vi "Parse NIC Info.vi"(6 "ifconfig":string="# This file describes the network interfaces available on your system\n# and how to activate them. For more information, see interfaces(5).\n\n# The loopback network interface\nauto lo\niface lo inet loopback\n\n# The primary network interface\n#auto eth0\n#iface eth0 inet dhcp\n# Example to keep MAC address between reboots\n#hwaddress ether DE:AD:BE:EF:CA:FE\n\n# The secondary network interface\n#auto eth1\n#iface eth1 inet dhcp\n\n# WiFi Example\n#auto wlan0\n#iface wlan0 inet dhcp\n#    wpa-ssid \"essid\"\n#    wpa-psk  \"password\"\n\n# Ethernet/RNDIS gadget (g_ether)\n# Used by: /opt/scripts/boot/autoconfigure_usb0.sh\niface usb0 inet static\n    address 192.168.7.2\n    netmask 255.255.255.252\n    network 192.168.7.0\n    gateway 192.168.7.1e", 8 "Error In":errorcluster, 9 "All NICs":string[](array[string]), 10 "interfaces config":string="# This file describes the network interfaces available on your system\n# and how to activate them. For more information, see interfaces(5).\n\n# The loopback network interface\nauto lo\niface lo inet loopback\n\n# The primary network interface\n#auto eth0\n#iface eth0 inet dhcp\n# Example to keep MAC address between reboots\n#hwaddress ether DE:AD:BE:EF:CA:FE\n\n# The secondary network interface\n#auto eth1\n#iface eth1 inet dhcp\n\n# WiFi Example\n#auto wlan0\n#iface wlan0 inet dhcp\n#    wpa-ssid \"essid\"\n#    wpa-psk  \"password\"\n\n# Ethernet/RNDIS gadget (g_ether)\n# Used by: /opt/scripts/boot/autoconfigure_usb0.sh\niface usb0 inet static\n    address 192.168.7.2\n    netmask 255.255.255.252\n    network 192.168.7.0\n    gateway 192.168.7.1e", 11 "Install LV Data":T1={"SSH Session"=refnum, "Status Log"="", "Detailed Log"="", "Credentials"={"Hostname or IP"="192.168.7.2", "Username"="root", "Password"=""}, "Target Info"={"OS Version"="", "CPU"="", "Systemd Version"="", "Internet Access"=FALSE, "Device Type"="", "LV Installed Ver"="", "LV Available Ver"="", "LV Upgrade Available"=FALSE, "Hostname"="", "NIC Info"=[]}, "Reboot Required?"=FALSE}) -> (0 "Error Out":errorcluster, 3 "Install LV Data":T1={"SSH Session"=refnum, "Status Log"="", "Detailed Log"="", "Credentials"={"Hostname or IP"="192.168.7.2", "Username"="root", "Password"=""}, "Target Info"={"OS Version"="", "CPU"="", "Systemd Version"="", "Internet Access"=FALSE, "Device Type"="", "LV Installed Ver"="", "LV Available Ver"="", "LV Upgrade Available"=FALSE, "Hostname"="", "NIC Info"=[]}, "Reboot Required?"=FALSE})   [LabVIEW 2014, in "LMH-LINX.lvlib"]
uses:
  <vilib>/MakerHub/LINX/LMH-LINX.lvlib
  <vilib>/MakerHub/LINX/Private/Utilties/Target Management/Install LV Data.ctl
  C:/Program Files (x86)/National Instruments/LabVIEW 2014/vi.lib/MakerHub/LINX/Resources/Renci.SshNet.dll
  Resources/Renci.SshNet.dll
  <vilib>/MakerHub/LINX/Private/Utilties/Target Management/Target Info.ctl
  <vilib>/MakerHub/LINX/Private/Utilties/Target Management/NIC Info.ctl
  <vilib>/MakerHub/LINX/Private/Utilties/Target Management/NIC Mode.ctl
  <vilib>/regexp/Match Regular Expression.xnode
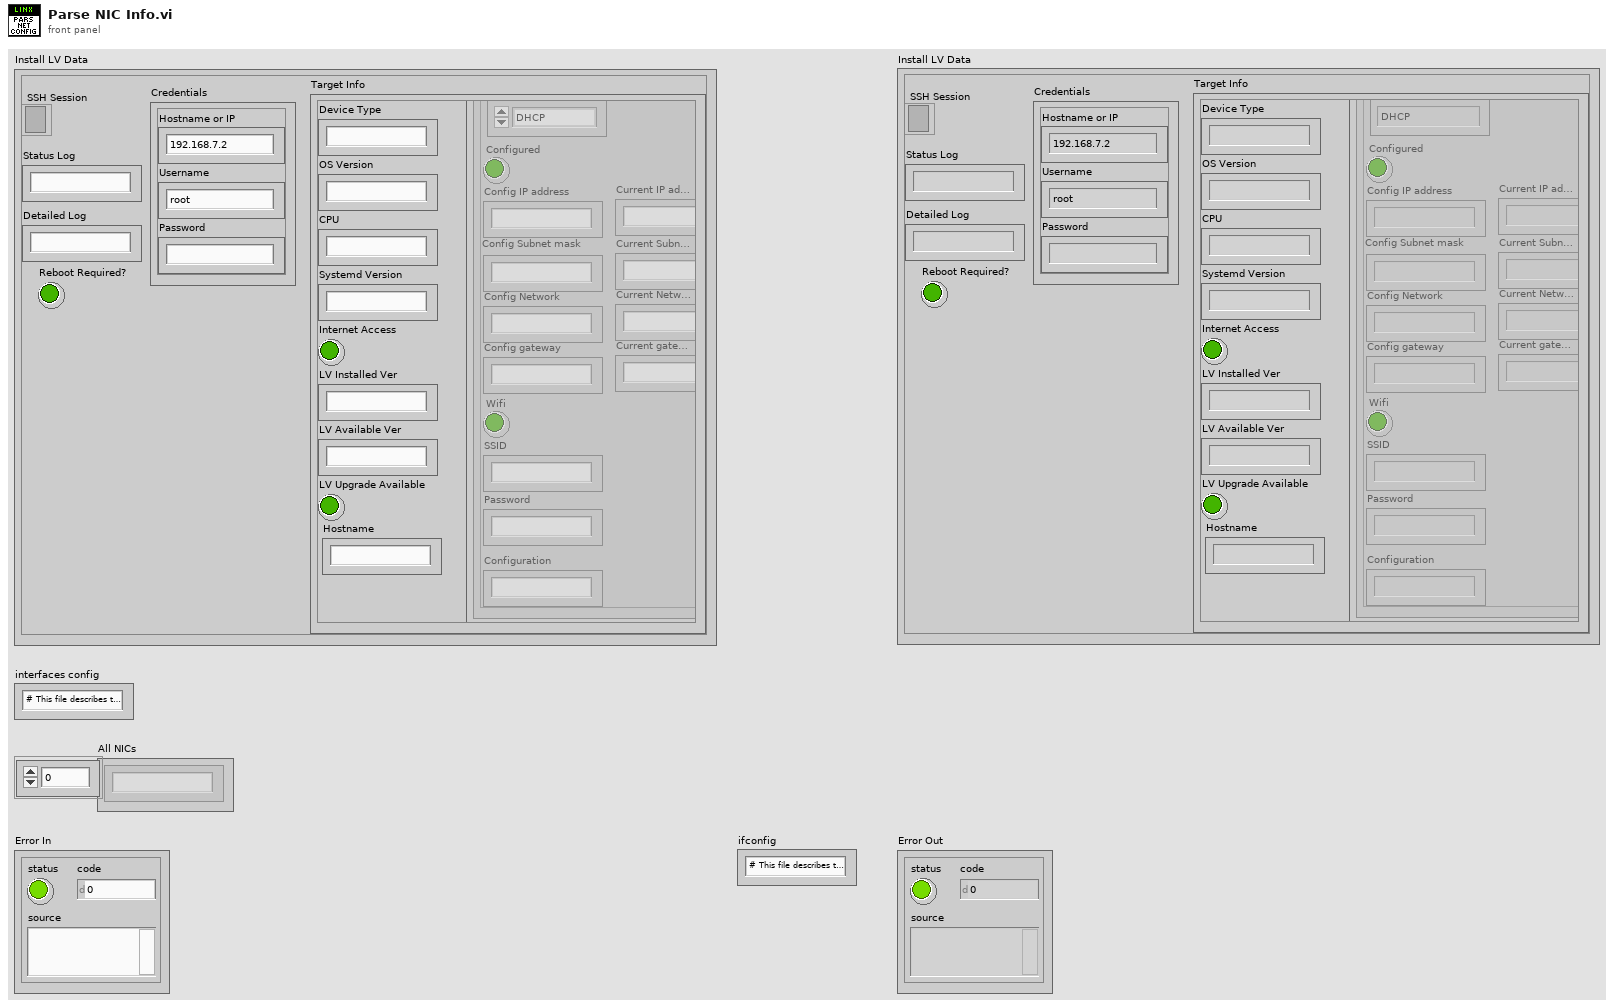
[diagram p1: front panel]
types:
  T1 = typedef "LMH-LINX.lvlib/Install LV Data.ctl" = cluster{"SSH Session":refnum<k24>, "Status Log":string, "Detailed Log":string, "Credentials":cluster{"Hostname or IP":string, "Username":string, "Password":string}, "Target Info":T2, "Reboot Required?":bool}
  T2 = typedef "LMH-LINX.lvlib/Target Info.ctl" = cluster{"OS Version":string, "CPU":string, "Systemd Version":string, "Internet Access":bool, "Device Type":string, "LV Installed Ver":string, "LV Available Ver":string, "LV Upgrade Available":bool, "Hostname":string, "NIC Info":T3[]}
  T3 = typedef "LMH-LINX.lvlib/NIC Info.ctl" = cluster{"Name":string, "NIC Mode":T4, "Configured":bool, "Config IP address":string, "Config Subnet mask":string, "Config Network":string, "Config gateway":string, "Wifi":bool, "SSID":string, "Password":string, "Configuration":string, "Current IP address":string, "Current Subnet mask":string, "Current gateway":string, "Current Network":string}
  T4 = typedef "LMH-LINX.lvlib/NIC Mode.ctl" = enum16{"DHCP", "Static", "Loopback"}
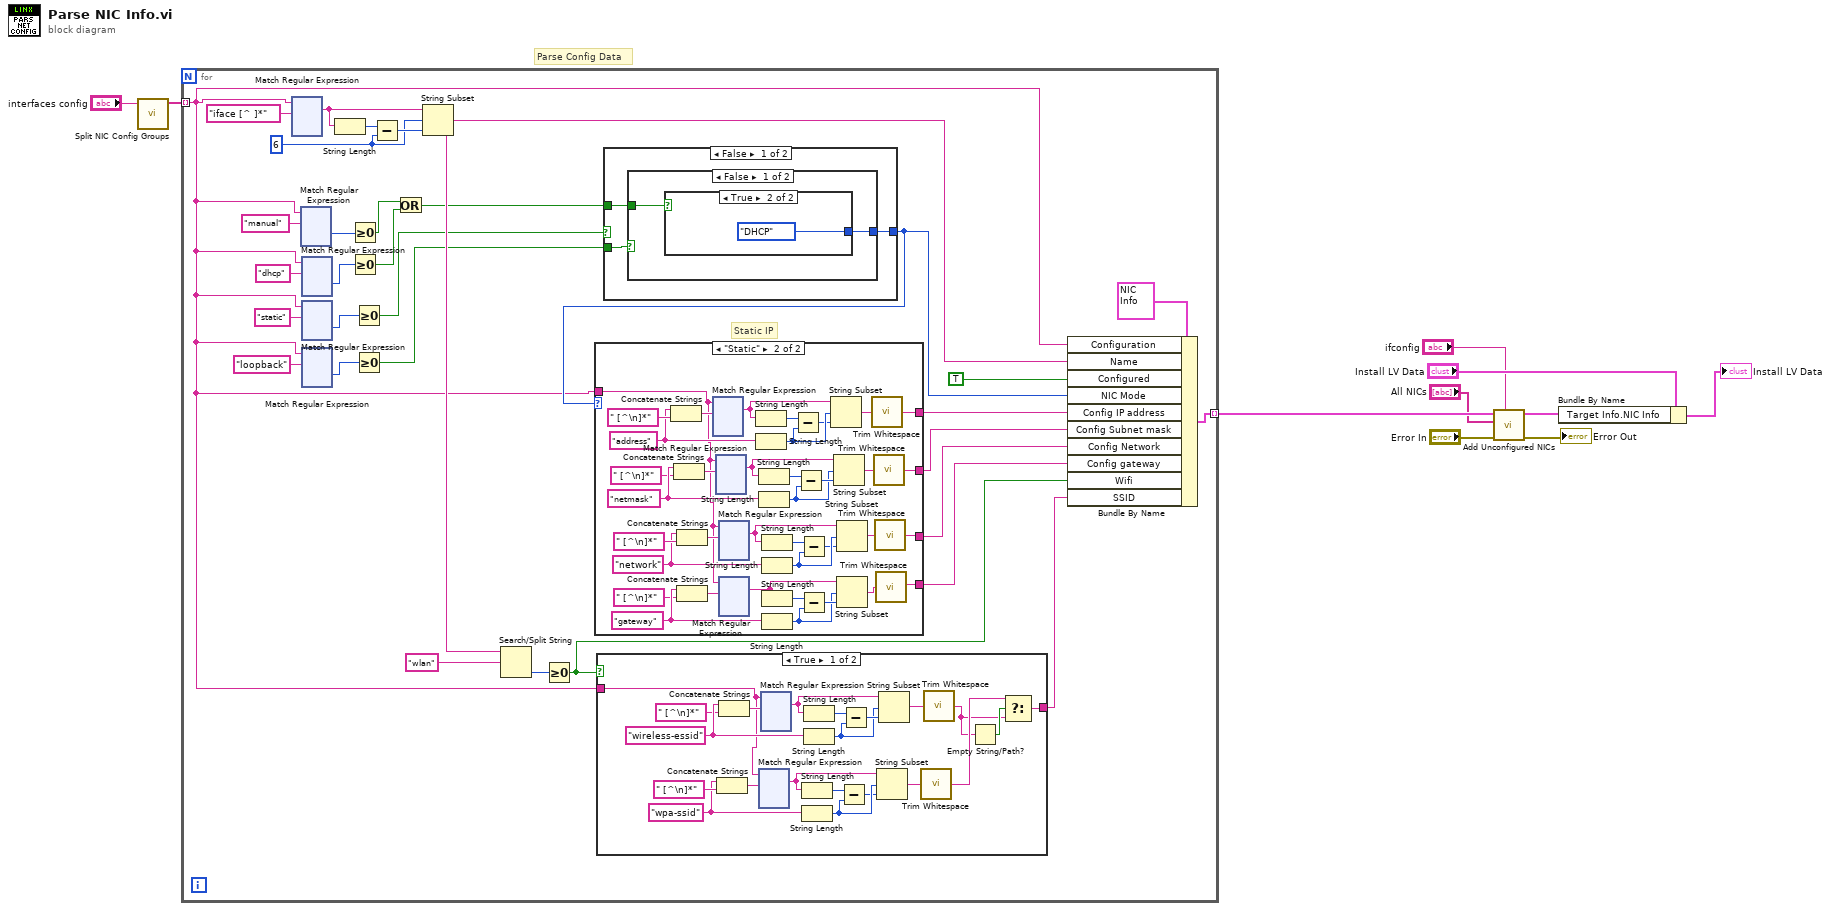
[diagram p0: block diagram]
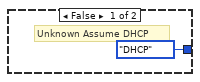
[diagram p2: hidden frame]
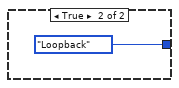
[diagram p3: hidden frame]
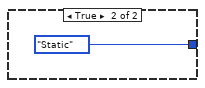
[diagram p4: hidden frame]
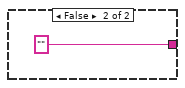
[diagram p5: hidden frame]
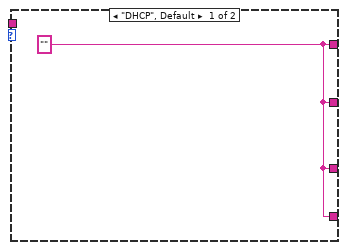
[diagram p6: hidden frame]
diagram:
  # "Parse Config Data"
  n1 = call <vilib>:"Split NIC Config Groups.vi"("Network Interface Config"="interfaces config") -> ("NIC Config Groups"=w9:string[])  [unwired: 10 in]
  n2 = for {
    tunnel: w9 -> [w12] mode=indexing
    tunnel: [w23] -> w6 mode=indexing
    w38 = 6 ("y")
    # "Static IP"
    n3 = xnode "Match Regular Expression"("input string"=w12, "regular expression"="iface [^ ]*") -> ("whole match"=w39:string)  [unwired: 4 in, 4 out]
    n4 = xnode "Match Regular Expression"("input string"=w12, "regular expression"="manual") -> ("offset past match"=w34:i32)  [unwired: 4 in, 4 out]
    n5 = xnode "Match Regular Expression"("input string"=w12, "regular expression"="dhcp") -> ("offset past match"=w32:i32)  [unwired: 4 in, 4 out]
    n6 = xnode "Match Regular Expression"("input string"=w12, "regular expression"="static") -> ("offset past match"=w33:i32)  [unwired: 4 in, 4 out]
    n7 = xnode "Match Regular Expression"("input string"=w12, "regular expression"="loopback") -> ("offset past match"=w20:i32)  [unwired: 4 in, 4 out]
    n8 = String Length(string=w39) -> (length=w41:i32)
    n9 = Greater Or Equal To 0?(x=w34) -> (x >= 0?=w16:bool)
    n10 = Greater Or Equal To 0?(x=w32) -> (x >= 0?=w15:bool)
    n11 = Greater Or Equal To 0?(x=w33) -> (x >= 0?=w18:bool)
    n12 = Greater Or Equal To 0?(x=w20) -> (x >= 0?=w17:bool)
    n13 = Subtract(x=w41, y=w38) -> (x-y=w40:i32)
    n14 = Or(x=w16, y=w15) -> (x .or. y?=w14:bool)
    n15 = String Subset(string=w39, offset (0)=w38, length (rest)=w40) -> (substring=w22:string)
    n16 = Search/Split String(string=w22, search string/char (-)="wlan") -> (offset of match=w25:i32)  [unwired: 1 in, 2 out]
    n17 = Greater Or Equal To 0?(x=w25) -> (x >= 0?=w24:bool)
    n18 = case shown="True" w24 {
      tunnel: w12 -> [w168 _]
      tunnel: [w165 "" ("whole match")] -> w11
      frame True {
        w173 = "wpa-ssid" ("string")
        w179 = "wireless-essid" ("string")
        n19 = Concatenate Strings(w173, " [^\n]*" ("regular expression")) -> (w174:string)
        n20 = Concatenate Strings(w179, " [^\n]*" ("regular expression")) -> (w178:string)
        n21 = xnode "Match Regular Expression"("input string"=w168, "regular expression"=w174) -> ("whole match"=w172:string)  [unwired: 4 in, 4 out]
        n22 = xnode "Match Regular Expression"("input string"=w168, "regular expression"=w178) -> ("whole match"=w180:string)  [unwired: 4 in, 4 out]
        n23 = String Length(string=w172) -> (length=w169:i32)
        n24 = String Length(string=w173) -> (length=w171:i32)
        n25 = String Length(string=w180) -> (length=w183:i32)
        n26 = String Length(string=w179) -> (length=w181:i32)
        n27 = Subtract(x=w169, y=w171) -> (x-y=w170:i32)
        n28 = Subtract(x=w183, y=w181) -> (x-y=w182:i32)
        n29 = String Subset(string=w172, offset (0)=w171, length (rest)=w170) -> (substring=w167:string)
        n30 = String Subset(string=w180, offset (0)=w181, length (rest)=w182) -> (substring=w176:string)
        n31 = call <vilib>:"Trim Whitespace.vi"("string"=w167) -> ("trimmed string"=w164:string)  [unwired: 1 in]
        n32 = call <vilib>:"Trim Whitespace.vi"("string"=w176) -> ("trimmed string"=w163:string)  [unwired: 1 in]
        n33 = Empty String/Path?(string/path=w163) -> (empty?=w166:bool)
        n34 = Select(t=w164, s=w166, f=w163) -> (s? t:f=w165:string)
      }
      frame False {
      }
    }
    n35 = case shown="False" w18 {
      tunnel: [w44 NIC_Mode."Static" ("NIC Mode")] -> w13
      tunnel: w17 -> [w45 _]
      tunnel: w14 -> [w43 _]
      frame False {
        n36 = case shown="False" w45 {
          tunnel: [w46 NIC_Mode."Loopback" ("NIC Mode")] -> w44
          tunnel: w43 -> [w47 _]
          frame False {
            n37 = case shown="True" w47 {
              tunnel: [NIC_Mode."DHCP" ("NIC Mode") NIC_Mode."DHCP" ("NIC Mode")] -> w46
              frame False {
                # "Unknown Assume DHCP"
              }
              frame True {
              }
            }
          }
          frame True {
          }
        }
      }
      frame True {
      }
    }
    n38 = case shown="\"Static\"" w13 {
      tunnel: w12 -> [_ w416]
      tunnel: [w407 w414] -> w30
      tunnel: [w407 w412] -> w29
      tunnel: [w407 w408] -> w28
      tunnel: [w407 w409] -> w27
      frame "DHCP", Default {
        w407 = "" ("whole match")
      }
      frame "Static" {
        w422 = "gateway" ("string")
        w429 = "network" ("string")
        w434 = "netmask" ("string")
        w442 = "address" ("string")
        n39 = Concatenate Strings(w442, " [^\n]*" ("regular expression")) -> (w443:string)
        n40 = Concatenate Strings(w434, " [^\n]*" ("regular expression")) -> (w433:string)
        n41 = Concatenate Strings(w429, " [^\n]*" ("regular expression")) -> (w430:string)
        n42 = Concatenate Strings(w422, " [^\n]*" ("regular expression")) -> (w421:string)
        n43 = xnode "Match Regular Expression"("input string"=w416, "regular expression"=w443) -> ("whole match"=w441:string)  [unwired: 4 in, 4 out]
        n44 = xnode "Match Regular Expression"("input string"=w416, "regular expression"=w433) -> ("whole match"=w419:string)  [unwired: 4 in, 4 out]
        n45 = xnode "Match Regular Expression"("input string"=w416, "regular expression"=w430) -> ("whole match"=w418:string)  [unwired: 4 in, 4 out]
        n46 = xnode "Match Regular Expression"("input string"=w416, "regular expression"=w421) -> ("whole match"=w417:string)  [unwired: 4 in, 4 out]
        n47 = String Length(string=w441) -> (length=w438:i32)
        n48 = String Length(string=w442) -> (length=w440:i32)
        n49 = String Length(string=w419) -> (length=w437:i32)
        n50 = String Length(string=w434) -> (length=w435:i32)
        n51 = String Length(string=w418) -> (length=w426:i32)
        n52 = String Length(string=w429) -> (length=w428:i32)
        n53 = String Length(string=w417) -> (length=w425:i32)
        n54 = String Length(string=w422) -> (length=w423:i32)
        n55 = Subtract(x=w438, y=w440) -> (x-y=w439:i32)
        n56 = Subtract(x=w437, y=w435) -> (x-y=w436:i32)
        n57 = Subtract(x=w426, y=w428) -> (x-y=w427:i32)
        n58 = Subtract(x=w425, y=w423) -> (x-y=w424:i32)
        n59 = String Subset(string=w441, offset (0)=w440, length (rest)=w439) -> (substring=w415:string)
        n60 = String Subset(string=w419, offset (0)=w435, length (rest)=w436) -> (substring=w413:string)
        n61 = String Subset(string=w418, offset (0)=w428, length (rest)=w427) -> (substring=w411:string)
        n62 = String Subset(string=w417, offset (0)=w423, length (rest)=w424) -> (substring=w410:string)
        n63 = call <vilib>:"Trim Whitespace.vi"("string"=w415) -> ("trimmed string"=w414:string)  [unwired: 1 in]
        n64 = call <vilib>:"Trim Whitespace.vi"("string"=w413) -> ("trimmed string"=w412:string)  [unwired: 1 in]
        n65 = call <vilib>:"Trim Whitespace.vi"("string"=w411) -> ("trimmed string"=w408:string)  [unwired: 1 in]
        n66 = call <vilib>:"Trim Whitespace.vi"("string"=w410) -> ("trimmed string"=w409:string)  [unwired: 1 in]
      }
    }
    n67 = Bundle By Name(cluster=T3 {"Name"="", "NIC Mode"=enum."DHCP", "Configured"=FALSE, "Config IP address"="", "Config Subnet mask"="", "Config Network"="", "Config gateway"="", "Wifi"=FALSE, "SSID"="", "Password"="", "Configuration"="", "Current IP address"="", "Current Subnet mask"="", "Current gateway"="", "Current Network"=""} ("NIC Info"), "Configuration"=w12, "Name"=w22, "Configured"=TRUE, "NIC Mode"=w13, "Config IP address"=w30, "Config Subnet mask"=w29, "Config Network"=w28, "Config gateway"=w27, "Wifi"=w24, "SSID"=w11) -> (w23:T3)
  }
  n68 = call <vilib>:"Add Unconfigured NICs.vi"("ifconfig"="ifconfig", "Error In"="Error In", "All NIC Names"="All NICs", "NIC Configs"=w6) -> ("Error Out"=→"Error Out":errorcluster, "NIC Configs"=w2:T3[])  [unwired: 6 in]
  n69 = Bundle By Name(cluster="Install LV Data", "Target Info.NIC Info"=w2) -> (→"Install LV Data":T1)
